vi "Set Node ID Map.vi"(8 "error in (no error)":errorcluster, 10 "Target IDs":map{string, T1}(c390), 11 "VolatusAPI in":refnum<class "VolatusAPI.lvclass">) -> (0 "error out":errorcluster, 3 "VolatusAPI out":refnum<class "VolatusAPI.lvclass">)   [LabVIEW 2020, in "Volatus.lvlib" / "VolatusAPI.lvclass"]
uses:
  VolatusAPI.lvclass
  VolatusAPI.lvclass/VolatusAPI.ctl
  Target Type.ctl
  Volatus.lvlib
  Target Info.ctl
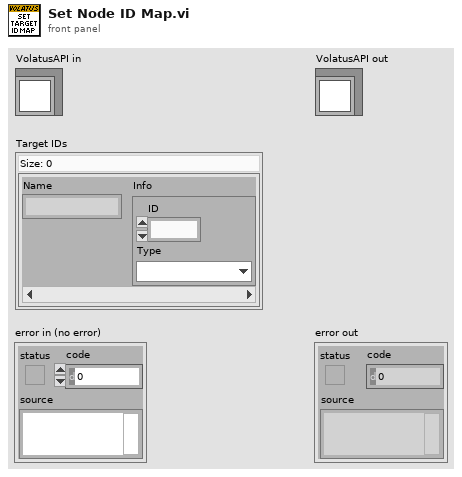
[diagram p1: front panel]
types:
  T1 = typedef "Volatus.lvlib/Target Info.ctl" = cluster{"ID":u32, "Type":T2}
  T2 = typedef "Volatus.lvlib/Target Type.ctl" = enum16{"Node", "Group"}
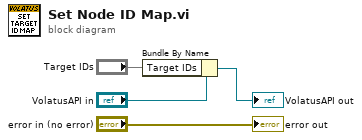
[diagram p0: block diagram]
diagram:
  n1 = Bundle By Name(cluster="VolatusAPI in", "Target IDs"="Target IDs") -> (→"VolatusAPI out":refnum<class "VolatusAPI.lvclass">)
  "error out" <- "error in (no error)"
